vi "Construct That Thang.vi"(8 "error in (no error)":errorcluster, 11 "Executioner in":refnum<class "Executioner.lvclass">) -> (0 "error out":errorcluster, 3 "iTest Step out":refnum<class "iTest Step.lvclass">)   [LabVIEW 2020, in "Test Executive.lvlib" / "Parallelizer Example.lvlib" / "iTest Step.lvclass"]
uses:
  <vilib>/gpm_packages/@cs/test-executive/Source/Sandbox/Parallelizer Example/iTest Step/iTest Step.lvclass
  <vilib>/gpm_packages/@cs/test-executive/Source/Test Executive/Executioner/Executioner.lvclass
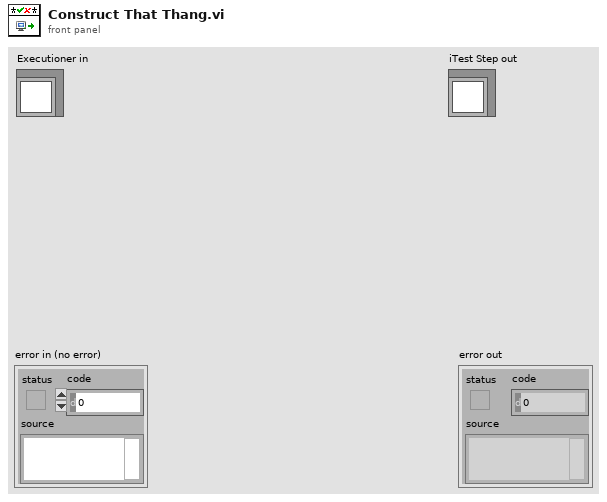
[diagram p1: front panel]
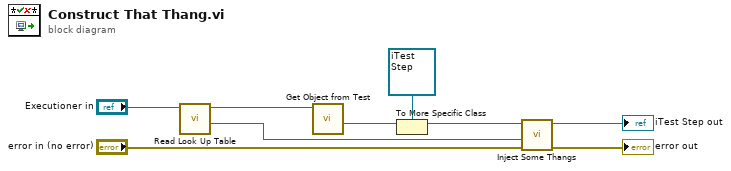
[diagram p0: block diagram]
diagram:
  n1 = call <vilib>:"Read Look Up Table.vi"("Executioner in"="Executioner in") -> ("Attributes Ref"=w1:refnum<data-value>, "Executioner out"=w9:refnum<class "Executioner.lvclass">)  [unwired: 9 in]
  n2 = call <vilib>:"Get Object from Test.vi"("Executioner in"=w9) -> ("Test"=w7:refnum<class>)  [unwired: 9 in, 1 out]
  n3 = To More Specific Class(target class=refnum<class "iTest Step.lvclass"> refnum ("iTest Step in"), reference=w7) -> (specific class reference=w5:refnum<class "iTest Step.lvclass">)  [unwired: 1 in, 1 out]
  n4 = call-dynamic "Inject Some Thangs.vi"("error in (no error)"="error in (no error)", "Attributes Ref"=w1, "iTest Step in"=w5) -> ("error out"=→"error out":errorcluster, "iTest Step out"=→"iTest Step out":refnum<class "iTest Step.lvclass">)  [unwired: 7 in]
